vi "libssh2_channel_get_exit_signal.vi"(8 "error in (no error)":errorcluster, 11 "channel":u64) -> (0 "error out":errorcluster, 1 "errmsg":string, 2 "exitsignal":string, 3 "return value":i32, 4 "langtag":string)   [LabVIEW 2013, in "libssh2.lvlib"]
uses:
  libssh2.lvlib
  libssh2.dll
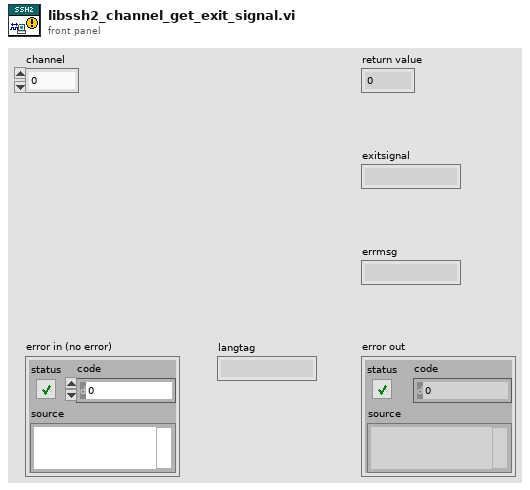
[diagram p1: front panel]
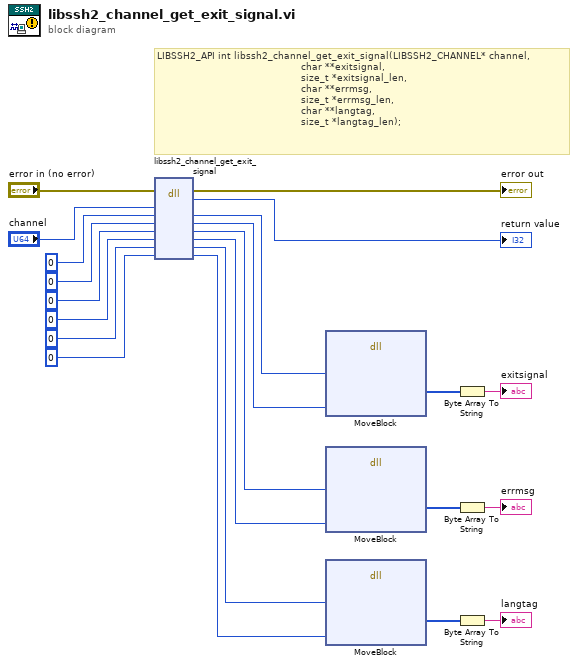
[diagram p0: block diagram]
diagram:
  # "LIBSSH2_API int libssh2_channel_get_exit_signal(LIBSSH2_CHANNEL* channel,\n                                                char **exitsignal,\n                                                size_t *exitsignal_len,\n                                                char **errmsg,\n                                                size_t *errmsg_len,\n                                                char **langtag,\n                                                size_t *langtag_len);"
  n1 = dll-call lib="C:/Users/pasca/source/repos/libssh2-labview/libssh2**.*" fn="libssh2_channel_get_exit_signal"(error in="error in (no error)", "channel"="channel", "exitsignal"=u64 0, "exitsignal_len"=i64 0, "errmsg"=u64 0, "errmsg_len"=i64 0, "langtag"=u64 0, "langtag_len"=i64 0) -> (error out=→"error out":errorcluster, "return value"=→"return value":i32, "exitsignal"=w13:u64, "exitsignal_len"=w12:i64, "errmsg"=w6:u64, "errmsg_len"=w5:i64, "langtag"=w2:u64, "langtag_len"=w1:i64)  [unwired: 3 in, 1 out]
  n2 = dll-call lib="LabVIEW" fn="MoveBlock"("ps"=w13, "size"=w12) -> ("pd"=w15:u8[])  [unwired: 7 in, 2 out]
  n3 = dll-call lib="LabVIEW" fn="MoveBlock"("ps"=w6, "size"=w5) -> ("pd"=w7:u8[])  [unwired: 7 in, 2 out]
  n4 = dll-call lib="LabVIEW" fn="MoveBlock"("ps"=w2, "size"=w1) -> ("pd"=w4:u8[])  [unwired: 7 in, 2 out]
  n5 = Byte Array To String(unsigned byte array=w15) -> (string=→"exitsignal":string)
  n6 = Byte Array To String(unsigned byte array=w7) -> (string=→"errmsg":string)
  n7 = Byte Array To String(unsigned byte array=w4) -> (string=→"langtag":string)
